vi "_TangoDeviceAttributesInfo.vi"(2 "error in":errorcluster, 3 "device name":string) -> (0 "error out":errorcluster, 1 "attributes_info":T5(array[cluster]))   [LabVIEW 2014, in "tango.lvlib"]
uses:
  tango.lvlib
  Common VIs/Typedefs/_AttributeAccess_t.ctl
  Common VIs/Typedefs/_AttributeFormat_t.ctl
  Common VIs/Typedefs/_TangoDataType_t.ctl
  Common VIs/Typedefs/_AttributeLevel_t.ctl
  tango_binding.so
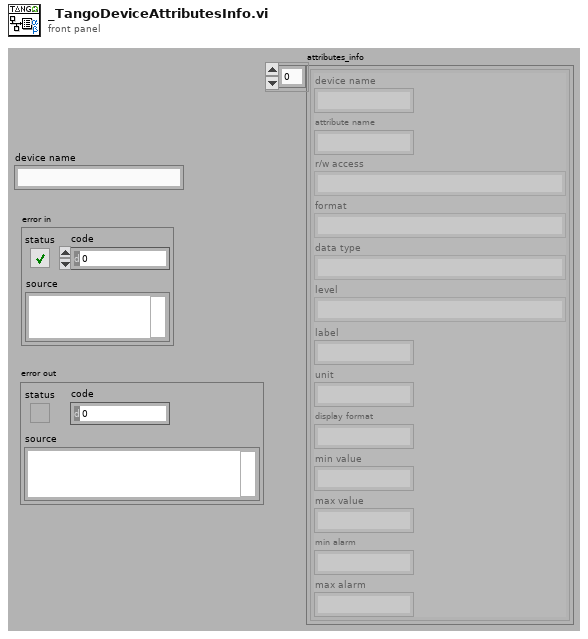
[diagram p1: front panel]
types:
  T1 = typedef "tango.lvlib/_AttributeAccess_t.ctl" = enum16{"READ", "READ_WITH_WRITE", "WRITE", "READ_WRITE", "UNKNOWN_ACCESS_TYPE"}
  T2 = typedef "tango.lvlib/_AttributeFormat_t.ctl" = enum16{"SCALAR", "SPECTRUM", "IMAGE", "UNKNOWN_FORMAT"}
  T3 = typedef "tango.lvlib/_TangoDataType_t.ctl" = enum16{"VOID", "BOOLEAN", "SHORT", "LONG", "FLOAT", "DOUBLE", "USHORT", "ULONG", "STRING", "CHAR_ARRAY", "SHORT_ARRAY", "LONG_ARRAY", "FLOAT_ARRAY", "DOUBLE_ARRAY", "USHORT_ARRAY", "ULONG_ARRAY", "STRING_ARRAY", "LONG_STRING_ARRAY", "DOUBLE_STRING_ARRAY", "STATE", "CONST_STRING", "BOOLEAN_ARRAY", "UCHAR", "LONG64", "ULONG64", "LONG64_ARRAY", "ULONG64_ARRAY", "INT (not supported)", "ENCODED (not supported)", "ENUM", "PIPE_BLOB (not supported)", "STATE_ARRAY", "UNKNOW_DATA_TYPE"}
  T4 = typedef "tango.lvlib/_AttributeLevel_t.ctl" = enum16{"OPERATOR", "EXPERT", "UNKNOWN_LEVEL"}
  T5 = cluster{"device name":string, "attribute name":string, "r/w access":T1, "format":T2, "data type":T3, "level":T4, "label":string, "unit":string, "display format":string, "min value":string, "max value":string, "min alarm":string, "max alarm":string}[]
  T6 = cluster{"device name":string, "attribute name":string, "r/w access":i16, "format":i16, "data type":i16, "level":i16, "label":string, "unit":string, "display format":string, "min value":string, "max value":string, "min alarm":string, "max alarm":string}
  T7 = cluster{"device name":string, "attribute name":string, "r/w access":i16, "format":i16, "data type":i16, "level":i16, "label":string, "unit":string, "display format":string, "min value":string, "max value":string, "min alarm":string, "max alarm":string}[]
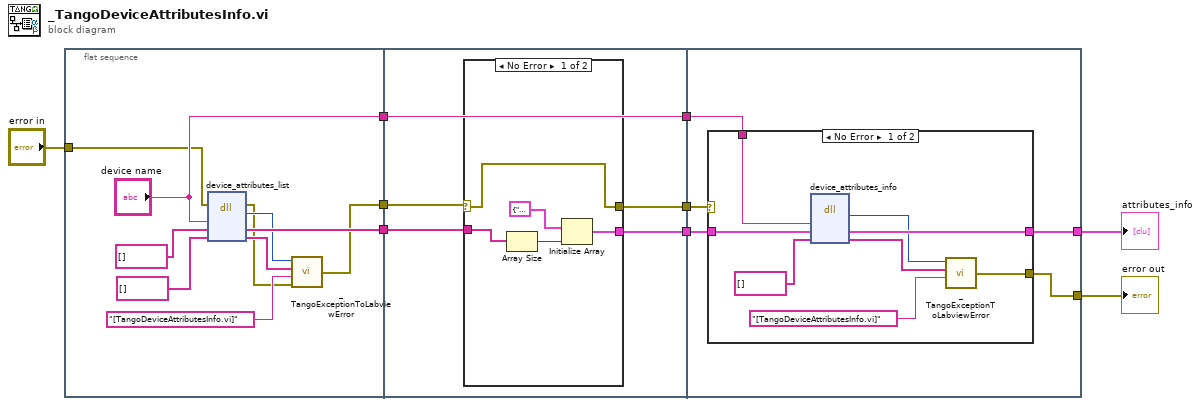
[diagram p0: block diagram]
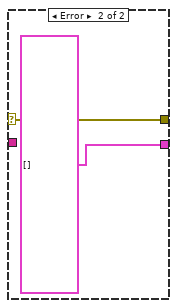
[diagram p2: hidden frame]
diagram:
  n1 = flat-sequence {
    tunnel: [w17] -> w9
    tunnel: ["device name"] -> w6
    tunnel: "error in" -> [w11]
    tunnel: [w12] -> w4
    tunnel: w9 -> [w24]
    tunnel: [w20] -> w8
    tunnel: [w23] -> w7
    tunnel: w6 -> [w23]
    tunnel: w4 -> [w22]
    tunnel: [w21] -> w3
    tunnel: w8 -> [w36]
    tunnel: w7 -> [w35]
    tunnel: w3 -> [w34]
    tunnel: [w33] -> w2
    tunnel: [w32] -> w1
    frame #0 {
      n2 = dll-call lib="tango_binding.*" fn="device_attributes_list"(error in=w11, "dev_name"="device name", "attributes_list"=string[] [] ("Error Stack"), "error_stack"=string[] [] ("Error Stack")) -> (error out=w10:errorcluster, "return type"=w15:i32, "attributes_list"=w17:string[], "error_stack"=w14:string[])  [unwired: 3 in, 1 out]
      n3 = call "_TangoExceptionToLabviewError.vi"("error in"=w10, "location"="[TangoDeviceAttributesInfo.vi]", "error stack"=w14, "error code"=w15) -> ("error out"=w12:errorcluster)
    }
    frame #1 {
      n4 = case shown="No Error" w22 {
        selector: w22 -> [w27 w31]
        tunnel: w24 -> [w29 _]
        tunnel: [w26 T7 []] -> w20
        tunnel: [w27 w31] -> w21
        frame No Error {
          n5 = Array Size(array=w29) -> (size(s)=w28:i32)
          n6 = Initialize Array(T6 {"device name"="", "attribute name"="", "r/w access"=0, "format"=0, "data type"=0, "level"=0, "label"="", "unit"="", "display format"="", "min value"="", "max value"="", "min alarm"="", "max alarm"=""} ("attribute info"), w28) -> (w26:T7)
        }
        frame Error {
        }
      }
    }
    frame #2 {
      n7 = case shown="No Error" w34 {
        selector: w34 -> [_ w46]
        tunnel: w36 -> [w43 w45]
        tunnel: [w42 w45] -> w32
        tunnel: w35 -> [w37 _]
        tunnel: [w38 w46] -> w33
        frame No Error {
          n8 = dll-call lib="tango_binding.*" fn="device_attributes_info"("dev_name"=w37, "attributes_info"=w43, "error_stack"=string[] [] ("Error Stack")) -> ("return type"=w39:i32, "attributes_info"=w42:T7, "error_stack"=w40:string[])  [unwired: 4 in, 2 out]
          n9 = call "_TangoExceptionToLabviewError.vi"("location"="[TangoDeviceAttributesInfo.vi]", "error stack"=w40, "error code"=w39) -> ("error out"=w38:errorcluster)  [unwired: 1 in]
        }
        frame Error {
        }
      }
    }
  }
  "error out" <- w2
  "attributes_info" <- w1
